vi "发送数据记录到文档(子VI).vi"(7 "错误输入":errorcluster, 9 "字符串":string="报文记录", 10 "数组":string[](array[string])) -> (0 "错误输出":errorcluster)   [LabVIEW 2016, in "潮位站数据传输.lvlib" / "TCP.lvclass"]
uses:
  TCP.lvclass
panel:
  out "路径":path
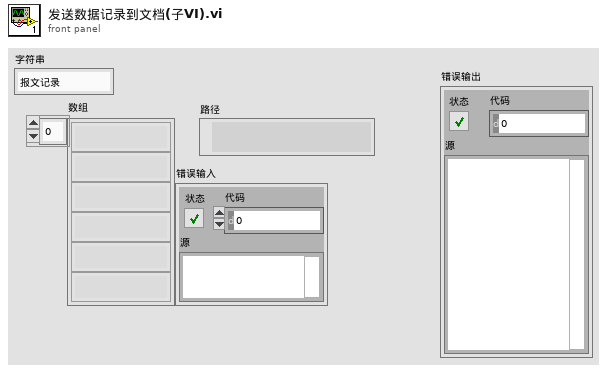
[diagram p1: front panel]
types:
  T1 = typedef "LVDateTimeRec.ctl" = cluster{"秒数的小数部分":dbl, "秒":i32, "分":i32, "时":i32, "日":i32, "月":i32, "年":i32, "天数（周）":i32, "天数（年）":i32, "DST":i32}
  T2 = enum16{"open", "replace", "create", "open or create", "replace or create", "replace or create with confirmation"}
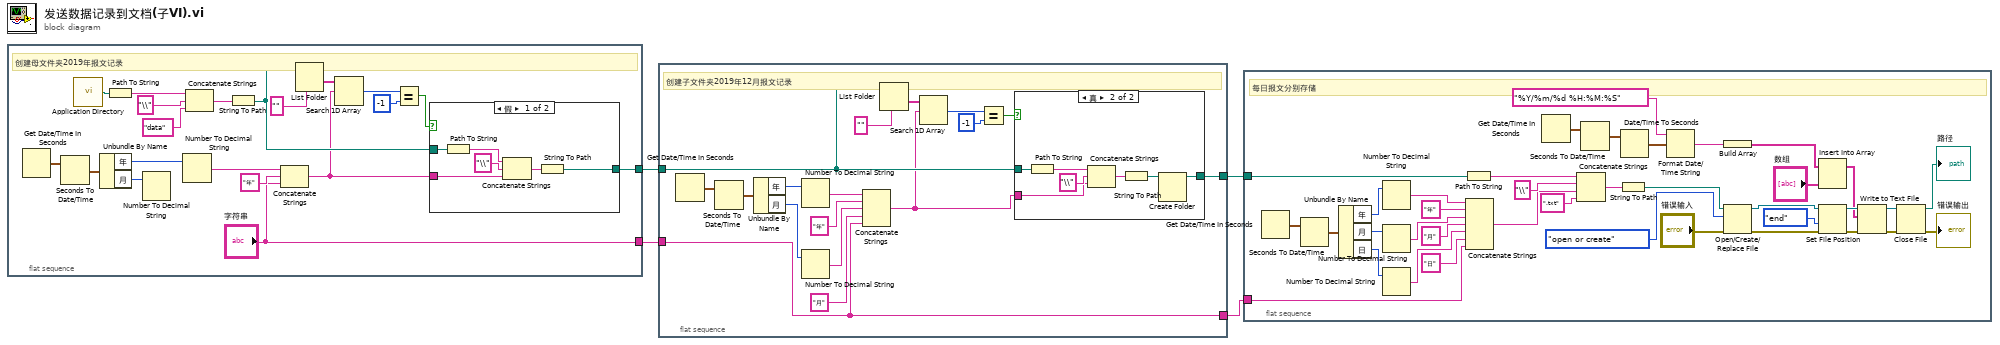
[diagram p0: block diagram]
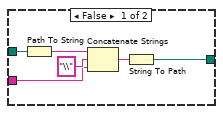
[diagram p2: hidden frame]
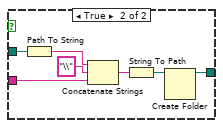
[diagram p3: hidden frame]
diagram:
  n1 = flat-sequence {
    tunnel: [w7] -> w4
    tunnel: ["字符串"] -> w2
    frame #0 {
      # "创建母文件夹2019年报文记录"
      n2 = Get Date/Time In Seconds() -> (seconds since 1Jan1904=w24:timestamp)
      n3 = Seconds To Date/Time(time stamp (now)=w24) -> (date time rec=w23:T1)  [unwired: 1 in]
      n4 = call <vilib>:"Application Directory.vi"() -> ("Application Directory"=w12:path)
      n5 = Unbundle By Name(w23) -> ("年"=w22:i32, "月"=w21:i32)
      n6 = Path To String(path=w12) -> (string=w15:string)
      n7 = Number To Decimal String(number=w21) -> ()  [unwired: 1 in, 1 out]
      n8 = Number To Decimal String(number=w22) -> (decimal integer string=w9:string)  [unwired: 1 in]
      n9 = Concatenate Strings(w15, "\\" ("字符串"), "data" ("名称或相对路径")) -> (w13:string)
      n10 = String To Path(string=w13) -> (path=w11:path)
      n11 = Concatenate Strings(w9, "年" ("字符串"), "字符串") -> (w8:string)
      n12 = List Folder(path=w11, pattern="" ("类型")) -> (folder names=w16:string[])  [unwired: 2 in, 3 out]
      n13 = Search 1D Array(1D array=w16, element=w8) -> (index of element=w20:i32)  [unwired: 1 in]
      n14 = Equal?(x=w20, y=-1) -> (x = y?=w18:bool)
      n15 = case shown="假" w18 {
        tunnel: w11 -> [w28 w36]
        tunnel: w8 -> [w27 w33]
        tunnel: [w26 w37] -> w7
        frame False {
          n16 = Path To String(path=w28) -> (string=w30:string)
          n17 = Concatenate Strings(w30, "\\" ("字符串"), w27) -> (w25:string)
          n18 = String To Path(string=w25) -> (path=w26:path)
        }
        frame True {
          n19 = Path To String(path=w36) -> (string=w35:string)
          n20 = Concatenate Strings(w35, "\\" ("字符串"), w33) -> (w31:string)
          n21 = String To Path(string=w31) -> (path=w32:path)
          n22 = Create Folder(path (use dialog)=w32) -> (created path=w37:path)  [unwired: 2 in, 2 out]
        }
      }
    }
  }
  n23 = flat-sequence {
    tunnel: w4 -> [w41]
    tunnel: [w39] -> w3
    tunnel: w2 -> [w38]
    tunnel: [w38] -> w1
    frame #0 {
      # "创建子文件夹2019年12月报文记录"
      n24 = Get Date/Time In Seconds() -> (seconds since 1Jan1904=w44:timestamp)
      n25 = Seconds To Date/Time(time stamp (now)=w44) -> (date time rec=w45:T1)  [unwired: 1 in]
      n26 = Unbundle By Name(w45) -> ("年"=w46:i32, "月"=w47:i32)
      n27 = Number To Decimal String(number=w46) -> (decimal integer string=w49:string)  [unwired: 1 in]
      n28 = Number To Decimal String(number=w47) -> (decimal integer string=w43:string)  [unwired: 1 in]
      n29 = Concatenate Strings(w49, "年" ("字符串"), w43, "月" ("字符串"), w38) -> (w40:string)
      n30 = List Folder(path=w41, pattern="" ("类型")) -> (folder names=w54:string[])  [unwired: 2 in, 3 out]
      n31 = Search 1D Array(1D array=w54, element=w40) -> (index of element=w50:i32)  [unwired: 1 in]
      n32 = Equal?(x=w50, y=-1) -> (x = y?=w52:bool)
      n33 = case shown="真" w52 {
        tunnel: w41 -> [w57 w66]
        tunnel: w40 -> [w56 w63]
        tunnel: [w55 w67] -> w39
        frame False {
          n34 = Path To String(path=w57) -> (string=w60:string)
          n35 = Concatenate Strings(w60, "\\" ("字符串"), w56) -> (w58:string)
          n36 = String To Path(string=w58) -> (path=w55:path)
        }
        frame True {
          n37 = Path To String(path=w66) -> (string=w65:string)
          n38 = Concatenate Strings(w65, "\\" ("字符串"), w63) -> (w62:string)
          n39 = String To Path(string=w62) -> (path=w61:path)
          n40 = Create Folder(path (use dialog)=w61) -> (created path=w67:path)  [unwired: 2 in, 2 out]
        }
      }
    }
  }
  n41 = flat-sequence {
    tunnel: w3 -> [w79]
    tunnel: w1 -> [w68]
    frame #0 {
      # "每日报文分别存储"
      n42 = Get Date/Time In Seconds() -> (seconds since 1Jan1904=w103:timestamp)
      n43 = Seconds To Date/Time(time stamp (now)=w103) -> (date time rec=w102:T1)  [unwired: 1 in]
      n44 = Unbundle By Name(w102) -> ("年"=w101:i32, "月"=w100:i32, "日"=w97:i32)
      n45 = Number To Decimal String(number=w101) -> (decimal integer string=w98:string)  [unwired: 1 in]
      n46 = Number To Decimal String(number=w100) -> (decimal integer string=w104:string)  [unwired: 1 in]
      n47 = Number To Decimal String(number=w97) -> (decimal integer string=w95:string)  [unwired: 1 in]
      n48 = Path To String(path=w79) -> (string=w87:string)
      n49 = Concatenate Strings(w98, "年" ("字符串"), w104, "月" ("字符串"), w95, "日" ("字符串"), w68) -> (w81:string)
      n50 = Get Date/Time In Seconds() -> (seconds since 1Jan1904=w71:timestamp)
      n51 = Concatenate Strings(w87, "\\" ("字符串"), w81, ".txt" ("字符串")) -> (w89:string)
      n52 = Seconds To Date/Time(time stamp (now)=w71) -> (date time rec=w74:T1)  [unwired: 1 in]
      n53 = String To Path(string=w89) -> (path=w85:path)
      n54 = Date/Time To Seconds(2:w74) -> (0:w72:timestamp)  [unwired: 1 in]
      n55 = Format Date/Time String(time format string (%c)="%Y/%m/%d %H:%M:%S" ("时间格式字符串(%c)"), seconds (now)=w72) -> (date/time string=w75:string)  [unwired: 1 in]
      n56 = Build Array(w75) -> (w70:string[])
      n57 = Open/Create/Replace File(file path (use dialog)=w85, error in="错误输入", operation (0:open)=T2."open or create" ("操作(0:open)")) -> (refnum out=w90:refnum<file>, error out=w91:errorcluster)  [unwired: 3 in, 1 out]
      n58 = Insert Into Array(array=w70, new element="数组") -> (w69:string[])  [unwired: 1 in]
      n59 = Set File Position(refnum=w90, from (0:start)=enum16{"start", "end", "current"}."end" ("自（0:起始）"), error in=w91) -> (refnum out=w92:refnum<file>, error out=w93:errorcluster)  [unwired: 1 in]
      n60 = Write to Text File(file (use dialog)=w92, text=w69, error in=w93) -> (refnum out=w84:refnum<file>, error out=w83:errorcluster)  [unwired: 1 in, 1 out]
      n61 = Close File(refnum=w84, error in=w83) -> (path=→"路径":path, error out=→"错误输出":errorcluster)
    }
  }
